vi "stopMotion.vi"(8 "error in (no error)":errorcluster, 11 "Model in":refnum<class "Model.lvclass">) -> (0 "error out":errorcluster, 3 "Model out":refnum<class "Model.lvclass">)   [LabVIEW 2013, in "Model.lvclass"]
uses:
  Model.lvclass
  Model.lvclass/Model.ctl
  <userlib>/Common/Devices/StepperMotor/StepperMotor/StepperMotor.lvclass/StepperMotor.ctl
  <userlib>/Common/Devices/StepperMotor/StepperMotor/StepperMotor.lvclass
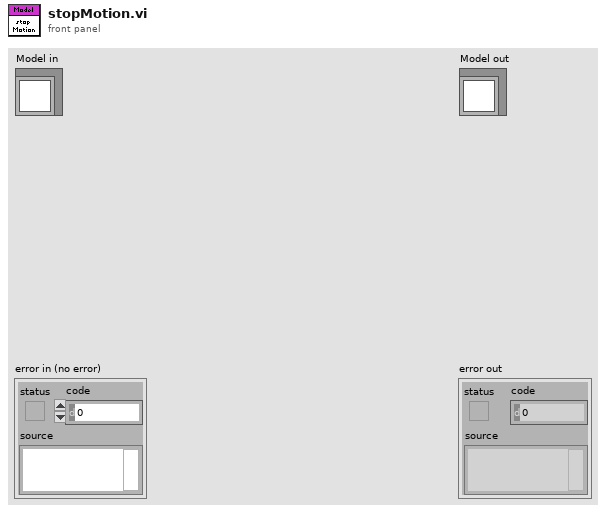
[diagram p1: front panel]
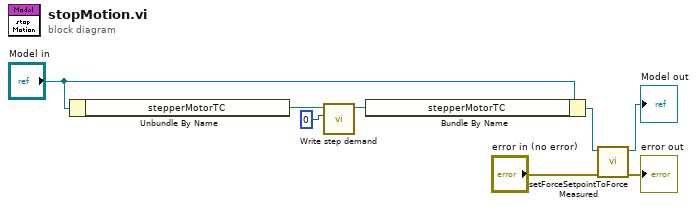
[diagram p0: block diagram]
diagram:
  n1 = Unbundle By Name("Model in") -> ("stepperMotorTC"=w6:refnum<class "StepperMotorTC.lvclass">)
  n2 = call <userlib>:"Write step demand.vi"("step demand"=i16 0, "StepperMotor in"=w6) -> ("StepperMotor out"=w5:refnum<class "StepperMotorTC.lvclass">)  [unwired: 9 in]
  n3 = Bundle By Name(cluster="Model in", "stepperMotorTC"=w5) -> (w4:refnum<class "Model.lvclass">)
  n4 = call "setForceSetpointToForceMeasured.vi"("error in (no error)"="error in (no error)", "Model in"=w4) -> ("error out"=→"error out":errorcluster, "Model out"=→"Model out":refnum<class "Model.lvclass">)  [unwired: 8 in]
